vi "set Active Object.vi"(10 "Active Object":i32, 11 "Scene in":refnum<class "Scene.lvclass">) -> (2 "Transform":T1, 3 "Scene out":refnum<class "Scene.lvclass">)   [LabVIEW 2022 SP3, in "Application.lvlib" / "Scene.lvclass"]
uses:
  Scene.lvclass
  Libraries/3D/Transform.ctl
  Libraries/3D/Vector 3D.ctl
  Scene.lvclass/Scene.ctl
  Libraries/3D/3D.lvlib
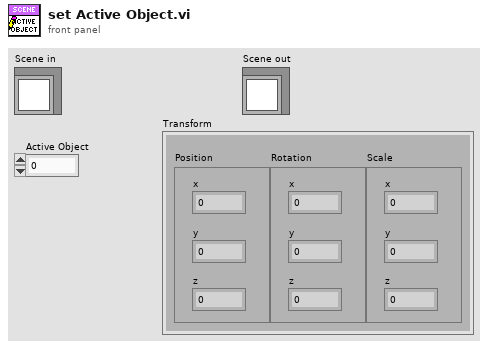
[diagram p1: front panel]
types:
  T1 = typedef "3D.lvlib/Transform.ctl" = cluster{"Position":T2, "Rotation":T2, "Scale":T2}
  T2 = typedef "3D.lvlib/Vector 3D.ctl" = cluster{"x":sgl, "y":sgl, "z":sgl}
  T3 = typedef "3D.lvlib/Object.ctl" = cluster{"Triangles":T4[], "Diffuse Colour":u32, "Transform":T1, "Name":string, "Enabled":bool, "Alpha":dbl}
  T4 = typedef "3D.lvlib/Triangle 3D.ctl" = cluster{"Point 1":T2, "Point 2":T2, "Point 3":T2}
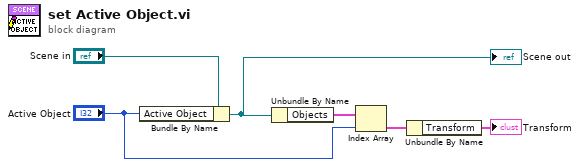
[diagram p0: block diagram]
diagram:
  n1 = Bundle By Name(cluster="Scene in", "Active Object"="Active Object") -> (w5:refnum<class "Scene.lvclass">)
  "Scene out" <- w5
  n2 = Unbundle By Name(w5) -> ("Objects"=w4:T3[])
  n3 = Index Array(array=w4, index="Active Object") -> (element=w2:T3)
  n4 = Unbundle By Name(w2) -> ("Transform"=→"Transform":T1)
